vi "calc pos to line.vi"(8 "error in (no error)":errorcluster, 10 "cursor pos":i32, 11 "String":string) -> (0 "error out":errorcluster, 3 "line num":i32)   [LabVIEW 2018, in "Data Parser.lvclass"]
uses:
  Data Parser.lvclass
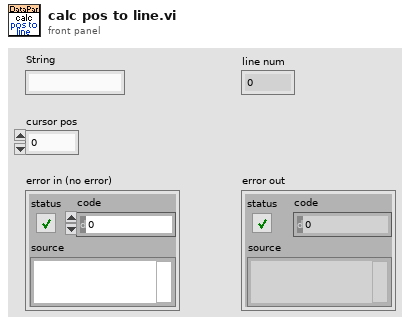
[diagram p1: front panel]
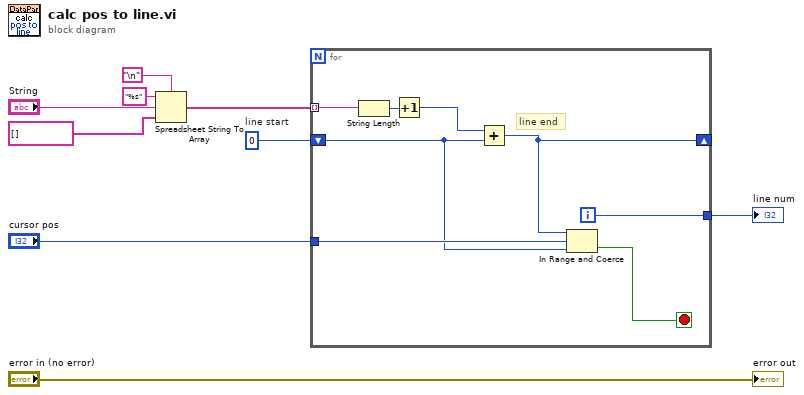
[diagram p0: block diagram]
diagram:
  w3 = 0  # line start
  n1 = Spreadsheet String To Array(delimiter (Tab)="\n", format string="%s", spreadsheet string="String", array type (2D Dbl)=string[] []) -> (array=w5:string[])
  n2 = for {
    tunnel: w5 -> [w17] mode=indexing
    tunnel: "cursor pos" -> [w14]
    shift-right: [w13] -> _
    shift-left: w3 -> [w12]
    tunnel: [w11] -> w2
    i -> [w11]
    stop <- w10 stop-if-true
    # "line end"
    n3 = String Length(string=w17) -> (length=w16:i32)
    n4 = Increment(x=w16) -> (x+1=w15:i32)
    n5 = Add(x=w15, y=w12) -> (x+y=w13:i32)
    n6 = In Range and Coerce(upper limit=w13, x=w14, lower limit=w12) -> (In Range?=w10:bool)  [unwired: 1 out]
  }
  "line num" <- w2
  "error out" <- "error in (no error)"
